vi "Sandbox.vi"() -> ()   [LabVIEW 2019]
uses:
  TypeDef/GUI Alarm customer settings.ctl
  <vilib>/addons/_JKI.lib/Serialization/JSON/JKI JSON Serialization.lvlib
panel:
  out "JSON String":string
  in  "GUI alarm customer settings":T1
  in  "error in (no error)":errorcluster
  # "Насос подачи масла"
  # "Насос очистки и охлаждения"
  # "Насос перекачки в бак подачи"
  # "Давление"
  # "Температура масла"
  # "Температура масла"
  # "Давление в камере"
  # "Давление в образце"
  # "Давление после насоса ВД"
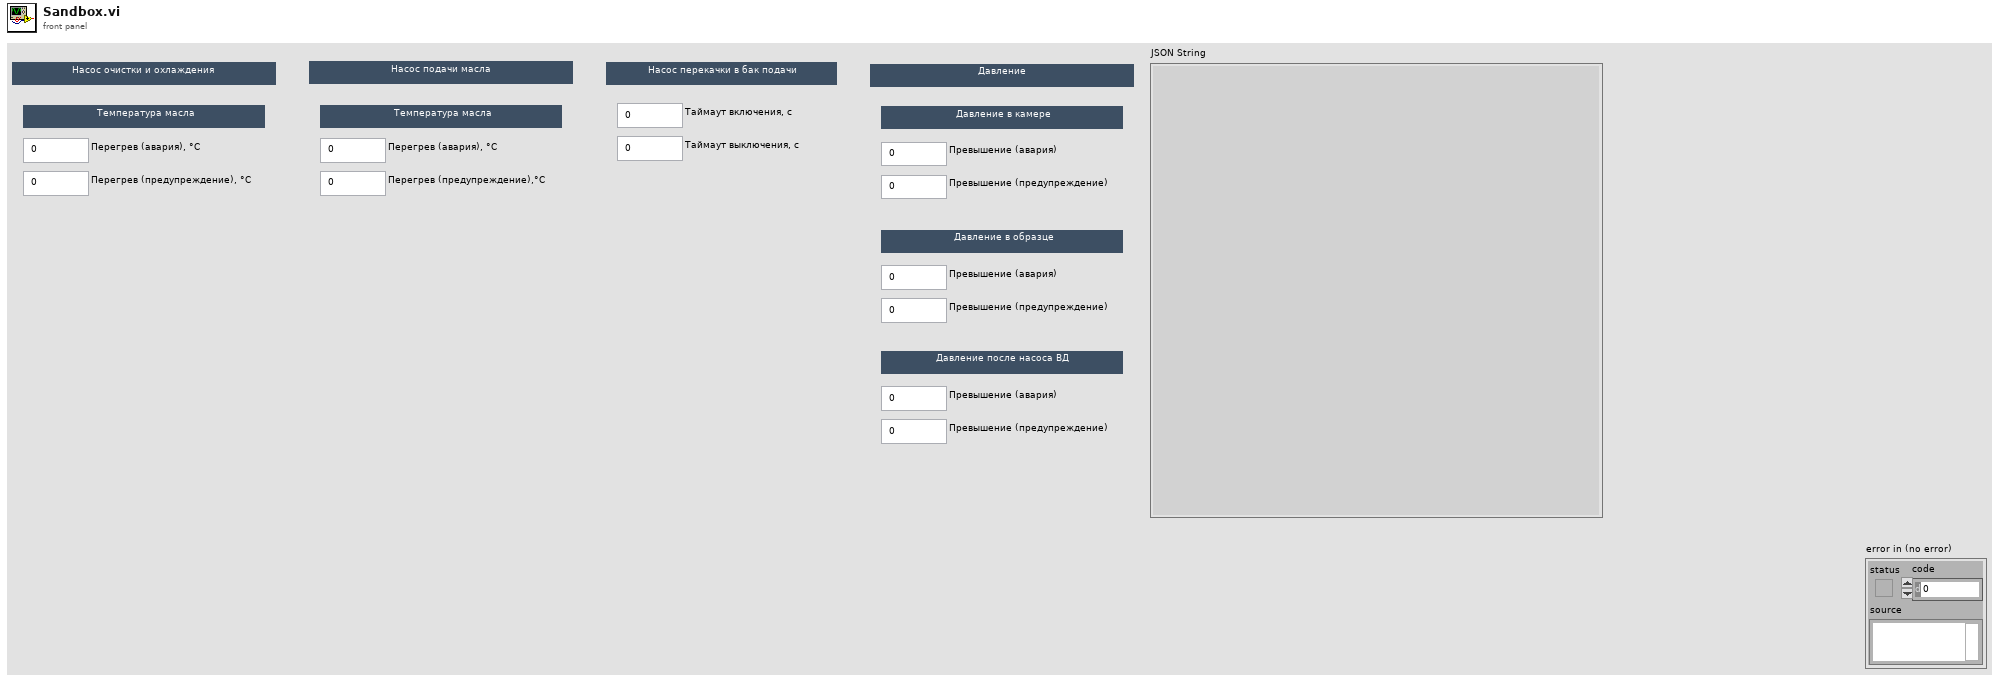
[diagram p1: front panel]
types:
  T1 = typedef "GUI Alarm customer settings.ctl" = cluster{"HIHI AI2":dbl, "HI AI2":dbl, "HIHI AI3":dbl, "HI AI3":dbl, "ENG0 OFF TIMEOUT":dbl, "ENG0 ON TIMEOUT":dbl, "HIHI AI7":dbl, "HI AI7":dbl, "HIHI AI6":dbl, "HI AI6":dbl, "HIHI AI5":dbl, "HI AI5":dbl}
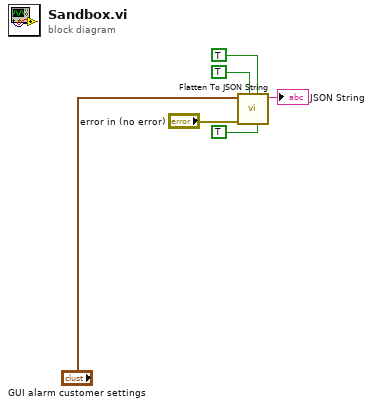
[diagram p0: block diagram]
diagram:
  n1 = call <vilib>:"Flatten To JSON String.vi"("Enums As String (F)"=TRUE, "Numeric Extensions (F)"=TRUE, "Multiline (T)"=TRUE, "error in (no error)"="error in (no error)", "Variant"="GUI alarm customer settings") -> ("JSON String"=→"JSON String":string)  [unwired: 5 in, 1 out]
